vi "E100Backup.vi"() -> ()   [LabVIEW 2012]
uses:
  <vilib>/Utility/NIReport.llb/NI_report.lvclass
  <vilib>/addons/database/Connection.llb/DB Tools Open Connec (Path).vi
  <vilib>/addons/database/Connection.llb/Conn Execute.vi
  <vilib>/addons/database/Recordset.llb/Rec Fetch Recordset Data (R).vi
  <vilib>/addons/database/Recordset.llb/Rec Destroy - Connection.vi
  <vilib>/Utility/NIReport.llb/Append Text Table to Report (wrap).vi
  <vilib>/addons/database/_DB Variant To Data/Database Variant To Data.xnode
  <vilib>/addons/database/NI_Database_API.lvlib
  <vilib>/Utility/NIReport.llb/Excel/NI_Excel.lvclass
  <vilib>/Utility/SMTP/NI_SMTPEmail.lvlib
panel:
  out "data 2":string
  out "data":string
  out "Value":variant
  in  "Table Control 3":string[][](table)
  out "appended array 4":string[](array[string])
  out "error out 5":errorcluster
  in  "Table Control 2":string[][](table)
  out "error out 4":errorcluster
  out "appended array 3":string[](array[string])
  out "recordset data 2":variant[][](array[variant])
  out "recordset data":variant[][](array[variant])
  out "appended array 2":string[](array[string])
  in  "Report Template":path=path "O:/Monitor/Report/E100Backup.xls"
  out "error out 2":errorcluster
  in  "Table Control":string[][](table)
  out "error out 3":errorcluster
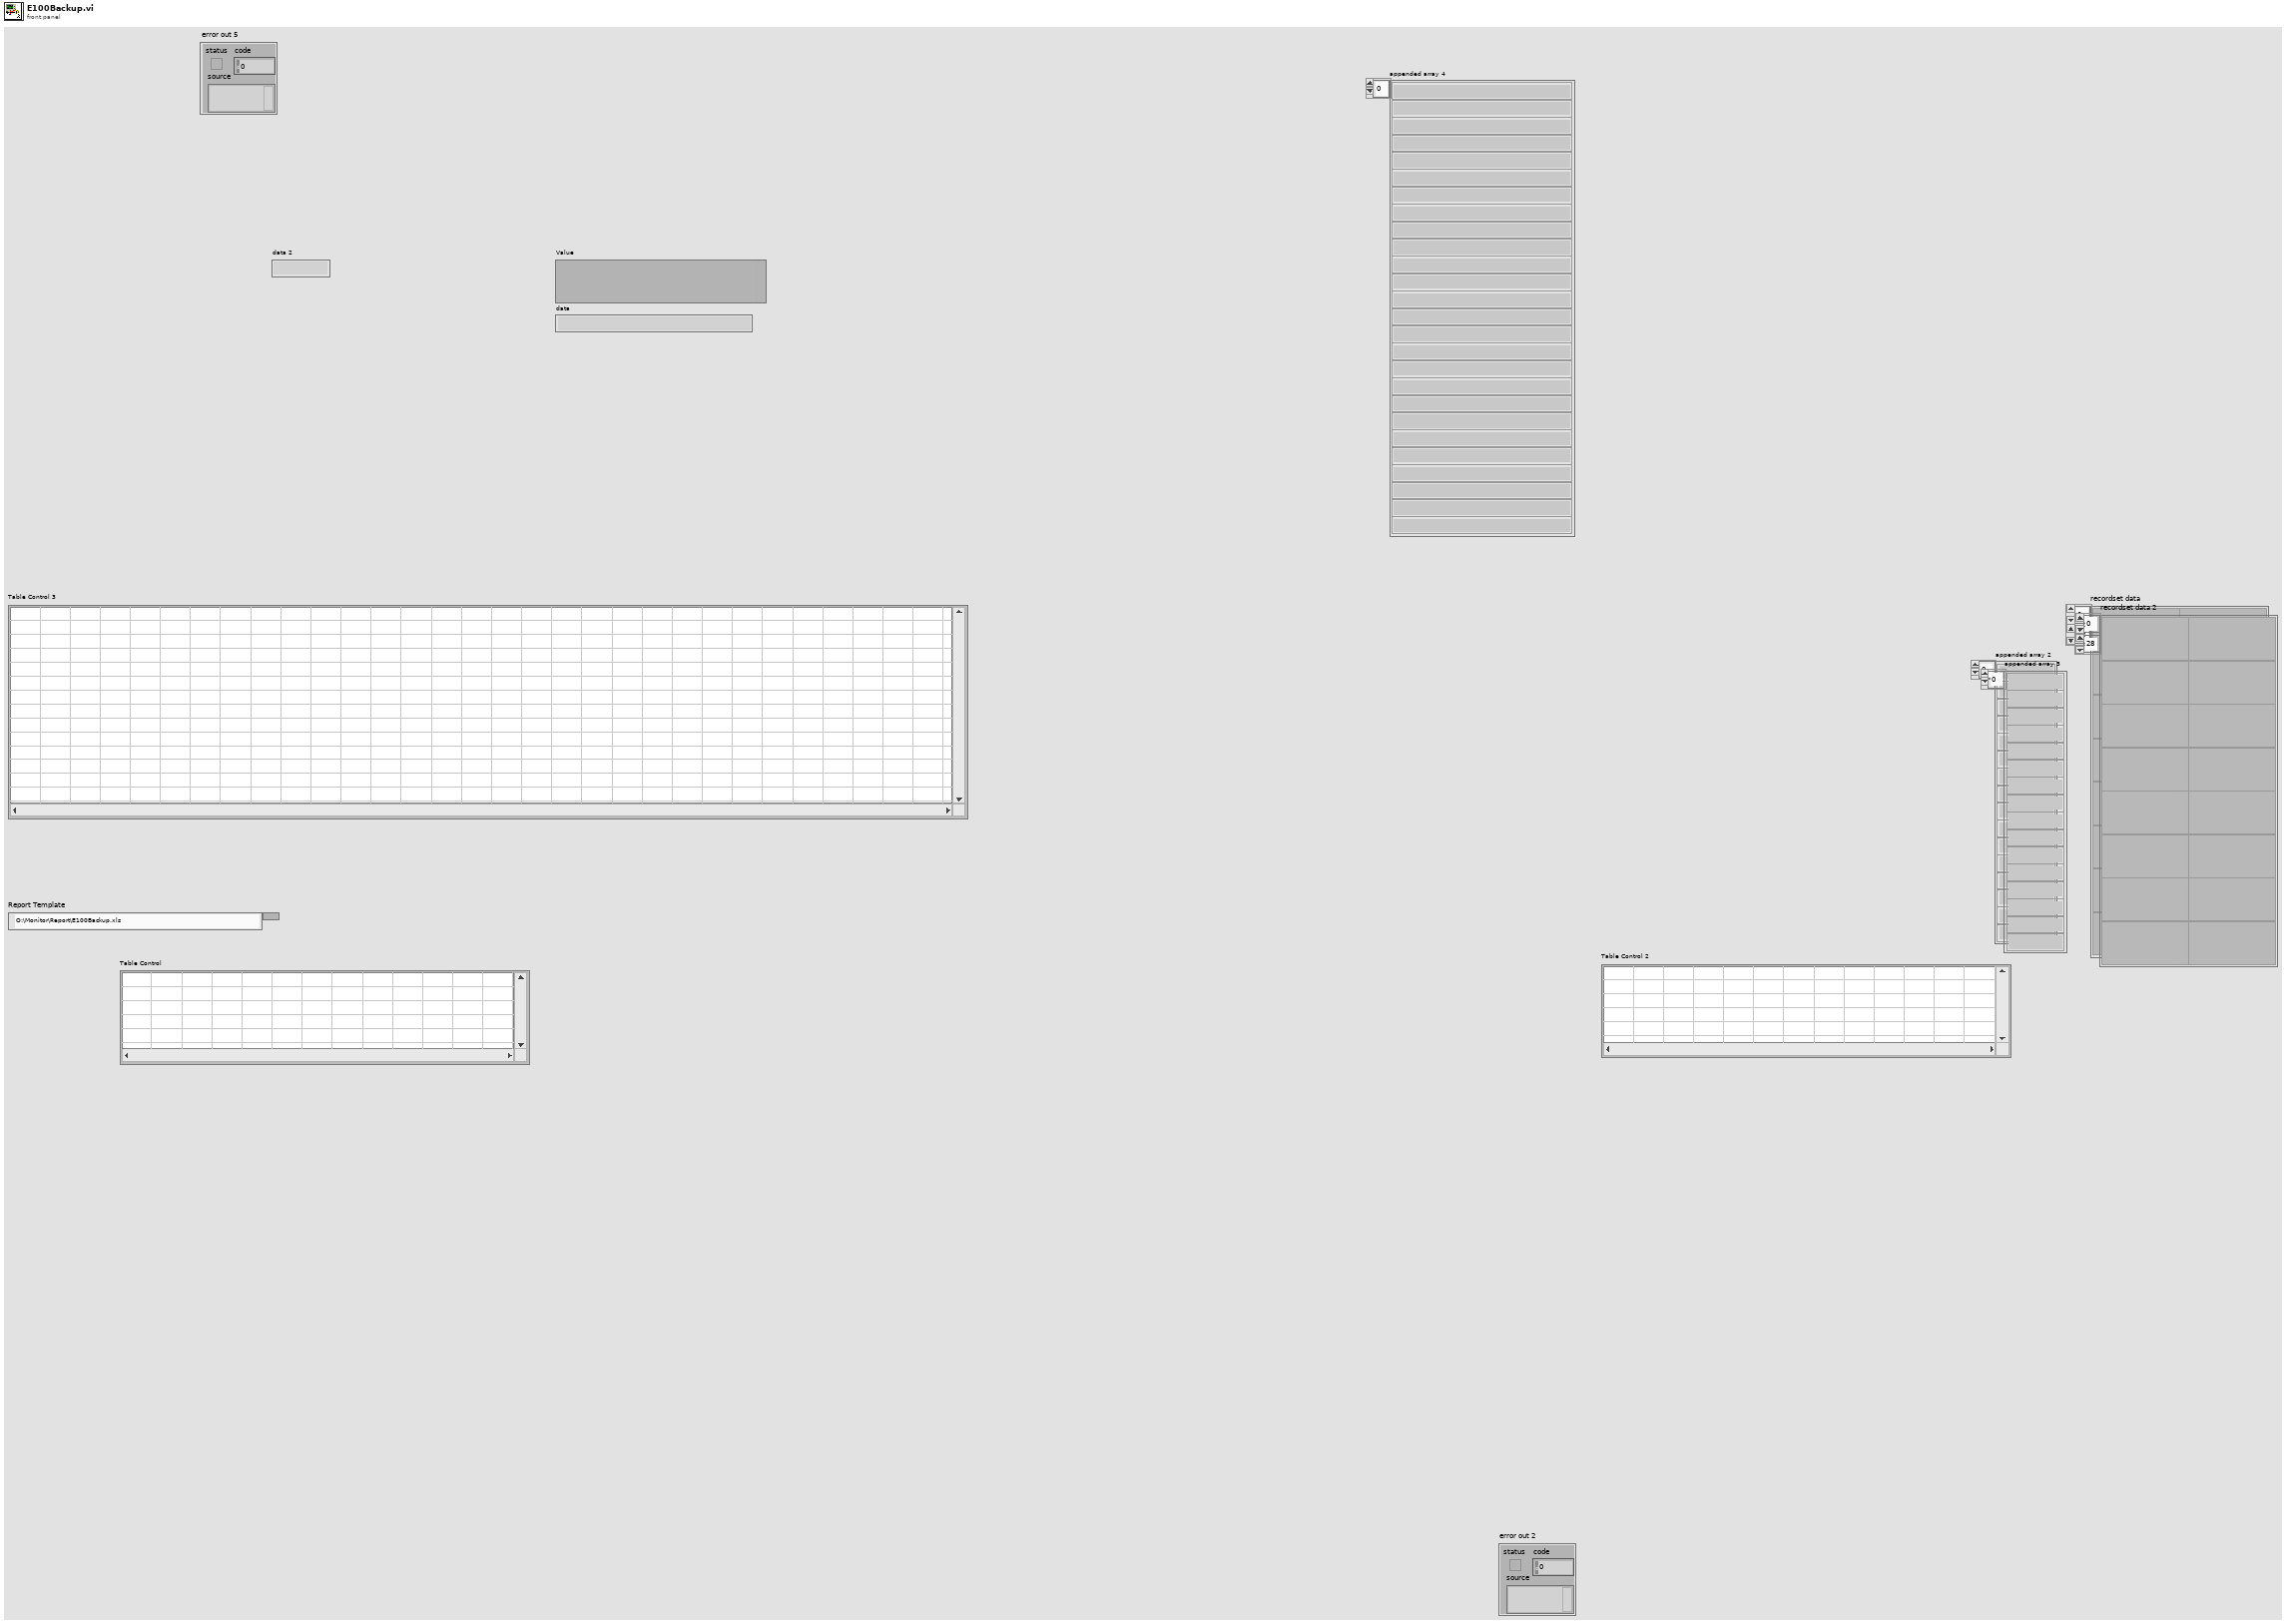
[diagram p1: front panel]
types:
  T1 = typedef "NI_Database_API.lvlib/Conn ObjectReference.ctl" = refnum<k1>
  T2 = typedef "NI_Database_API.lvlib/Rec ObjectReference.ctl" = refnum<k1>
  T3 = enum16{"Standard Report", "HTML", "Word", "Excel"}
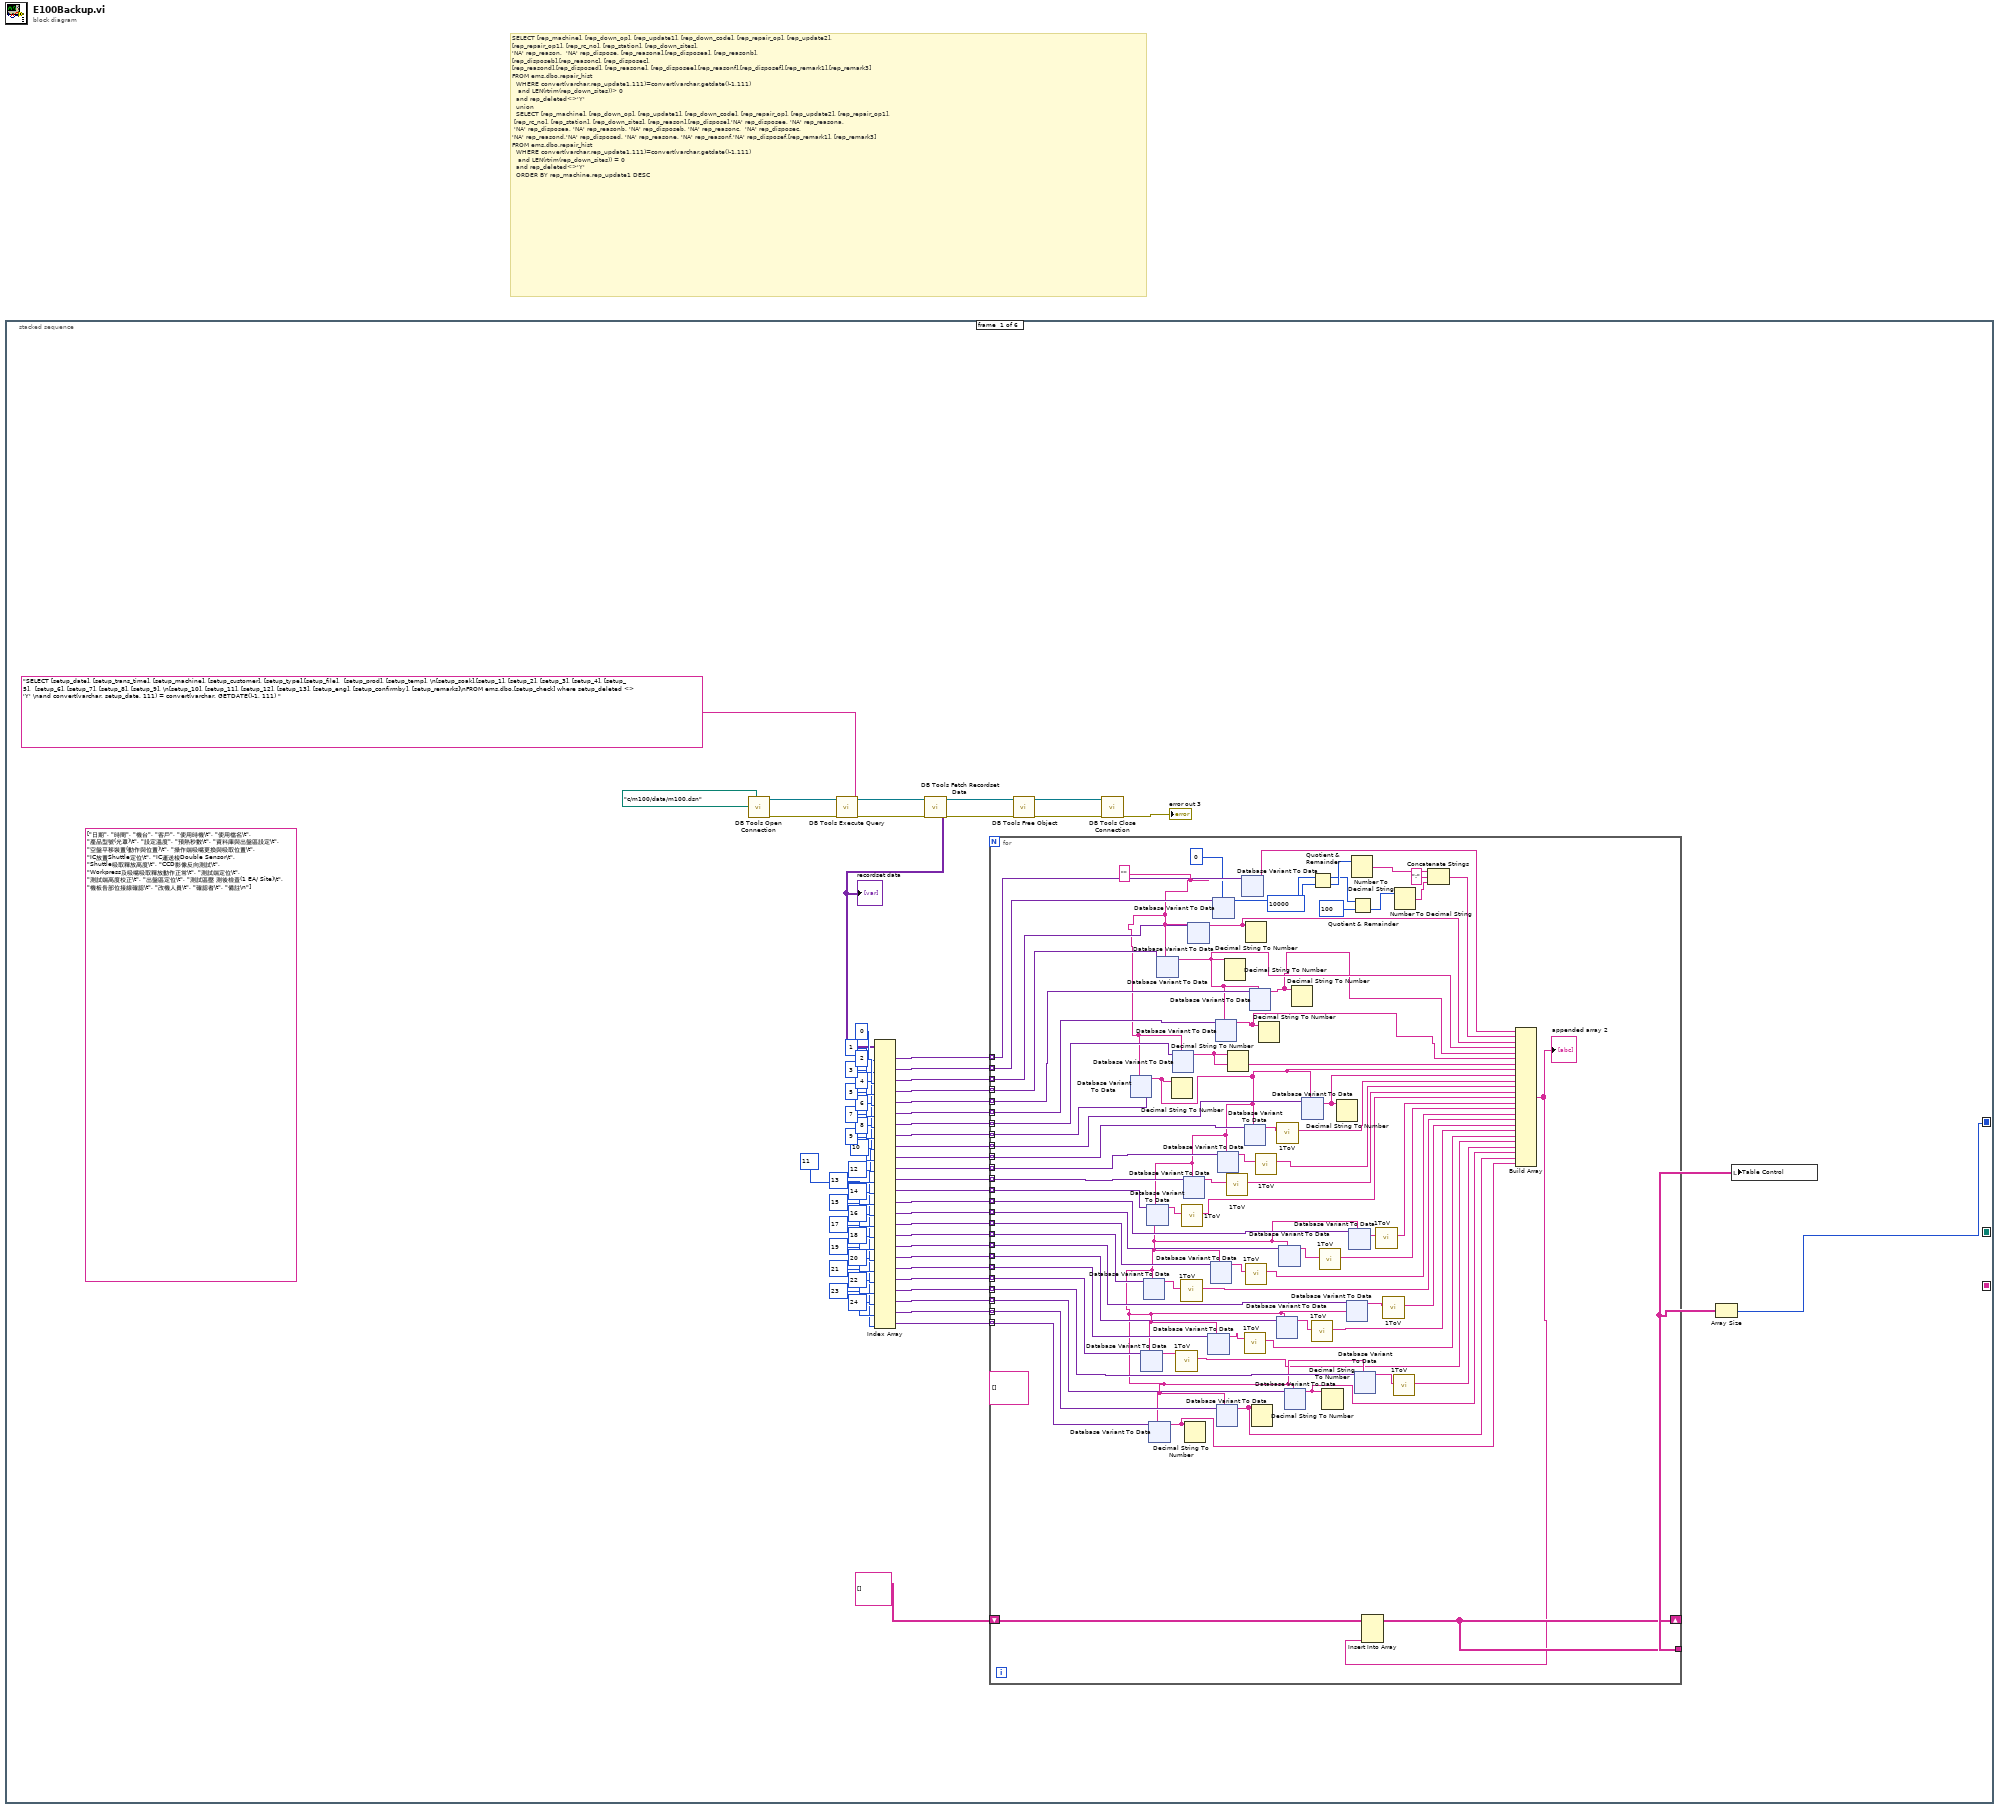
[diagram p0: block diagram]
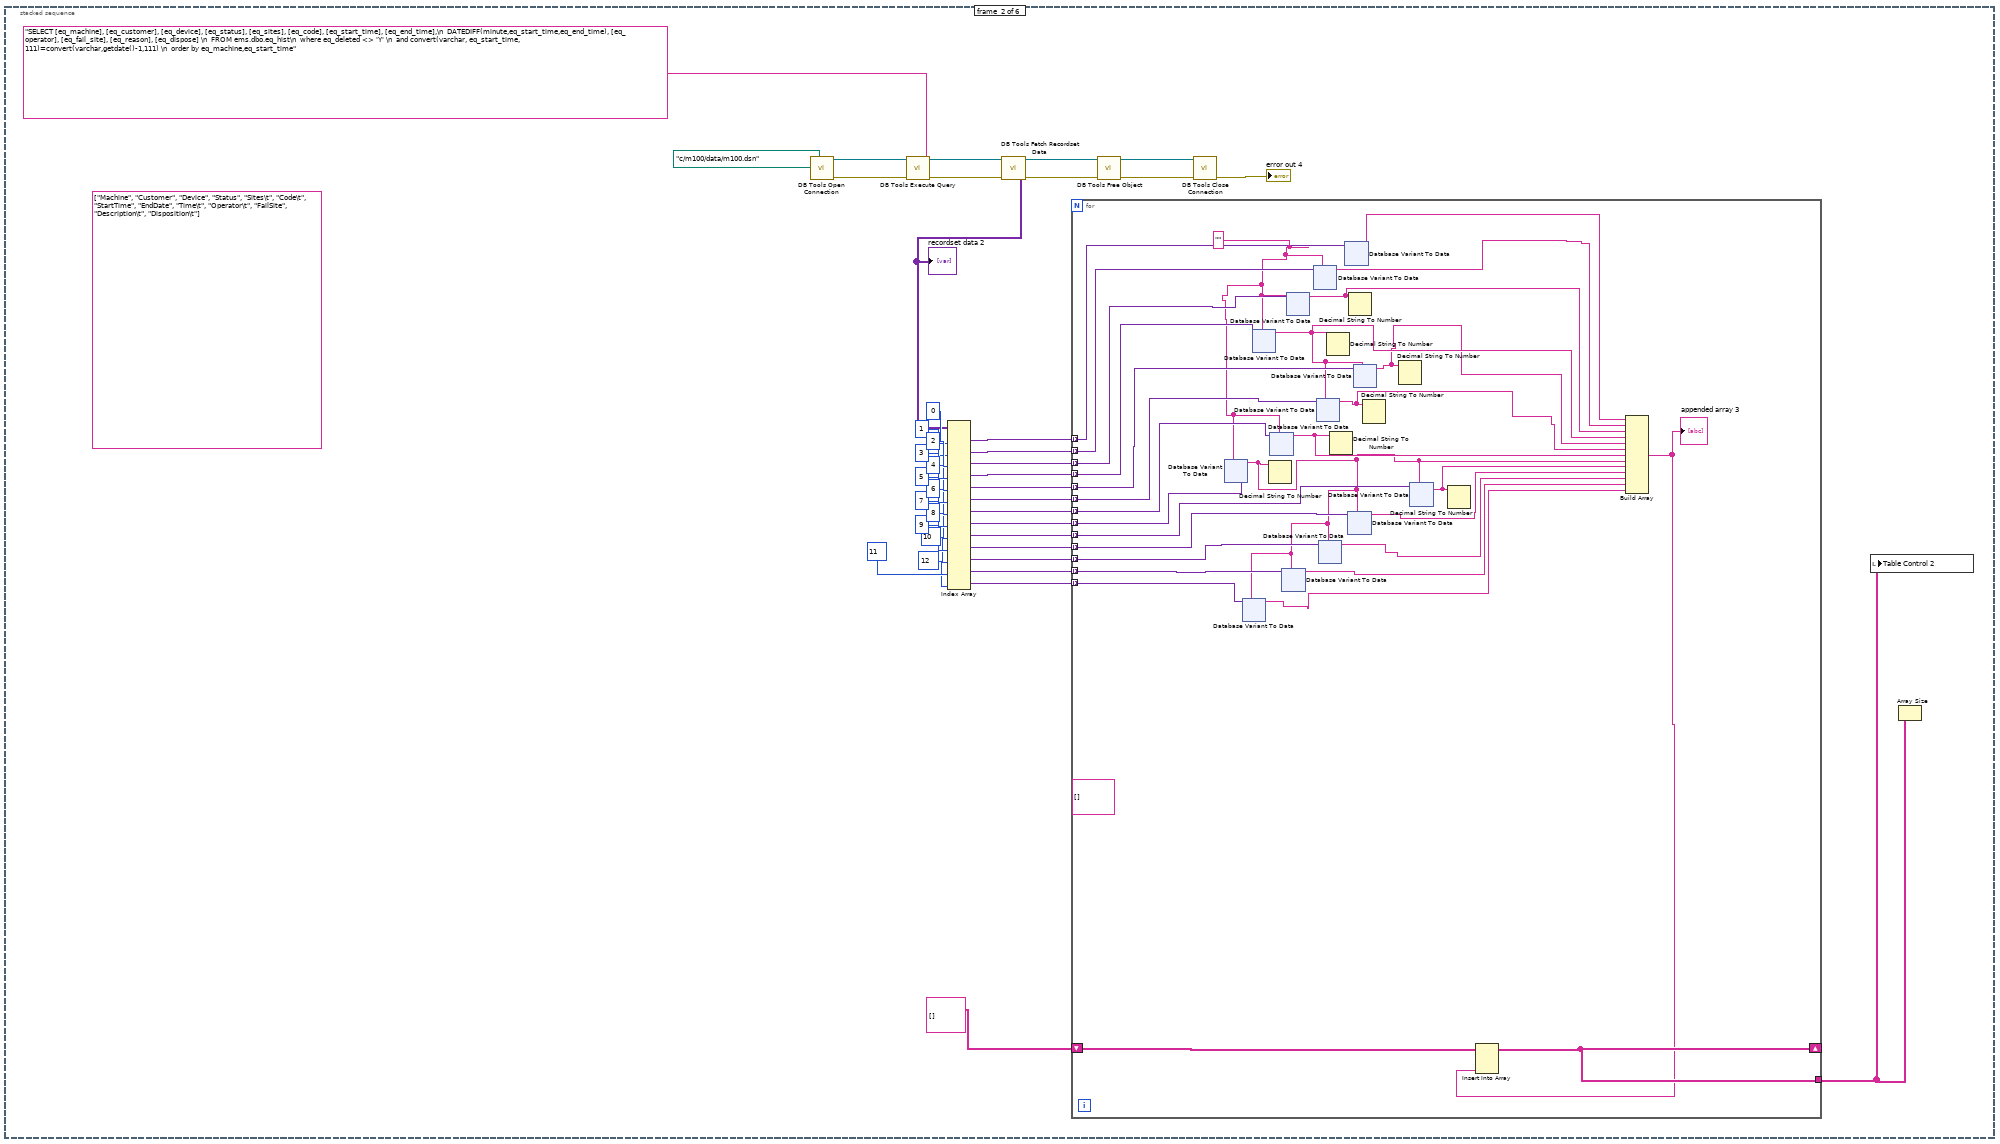
[diagram p2: hidden frame]
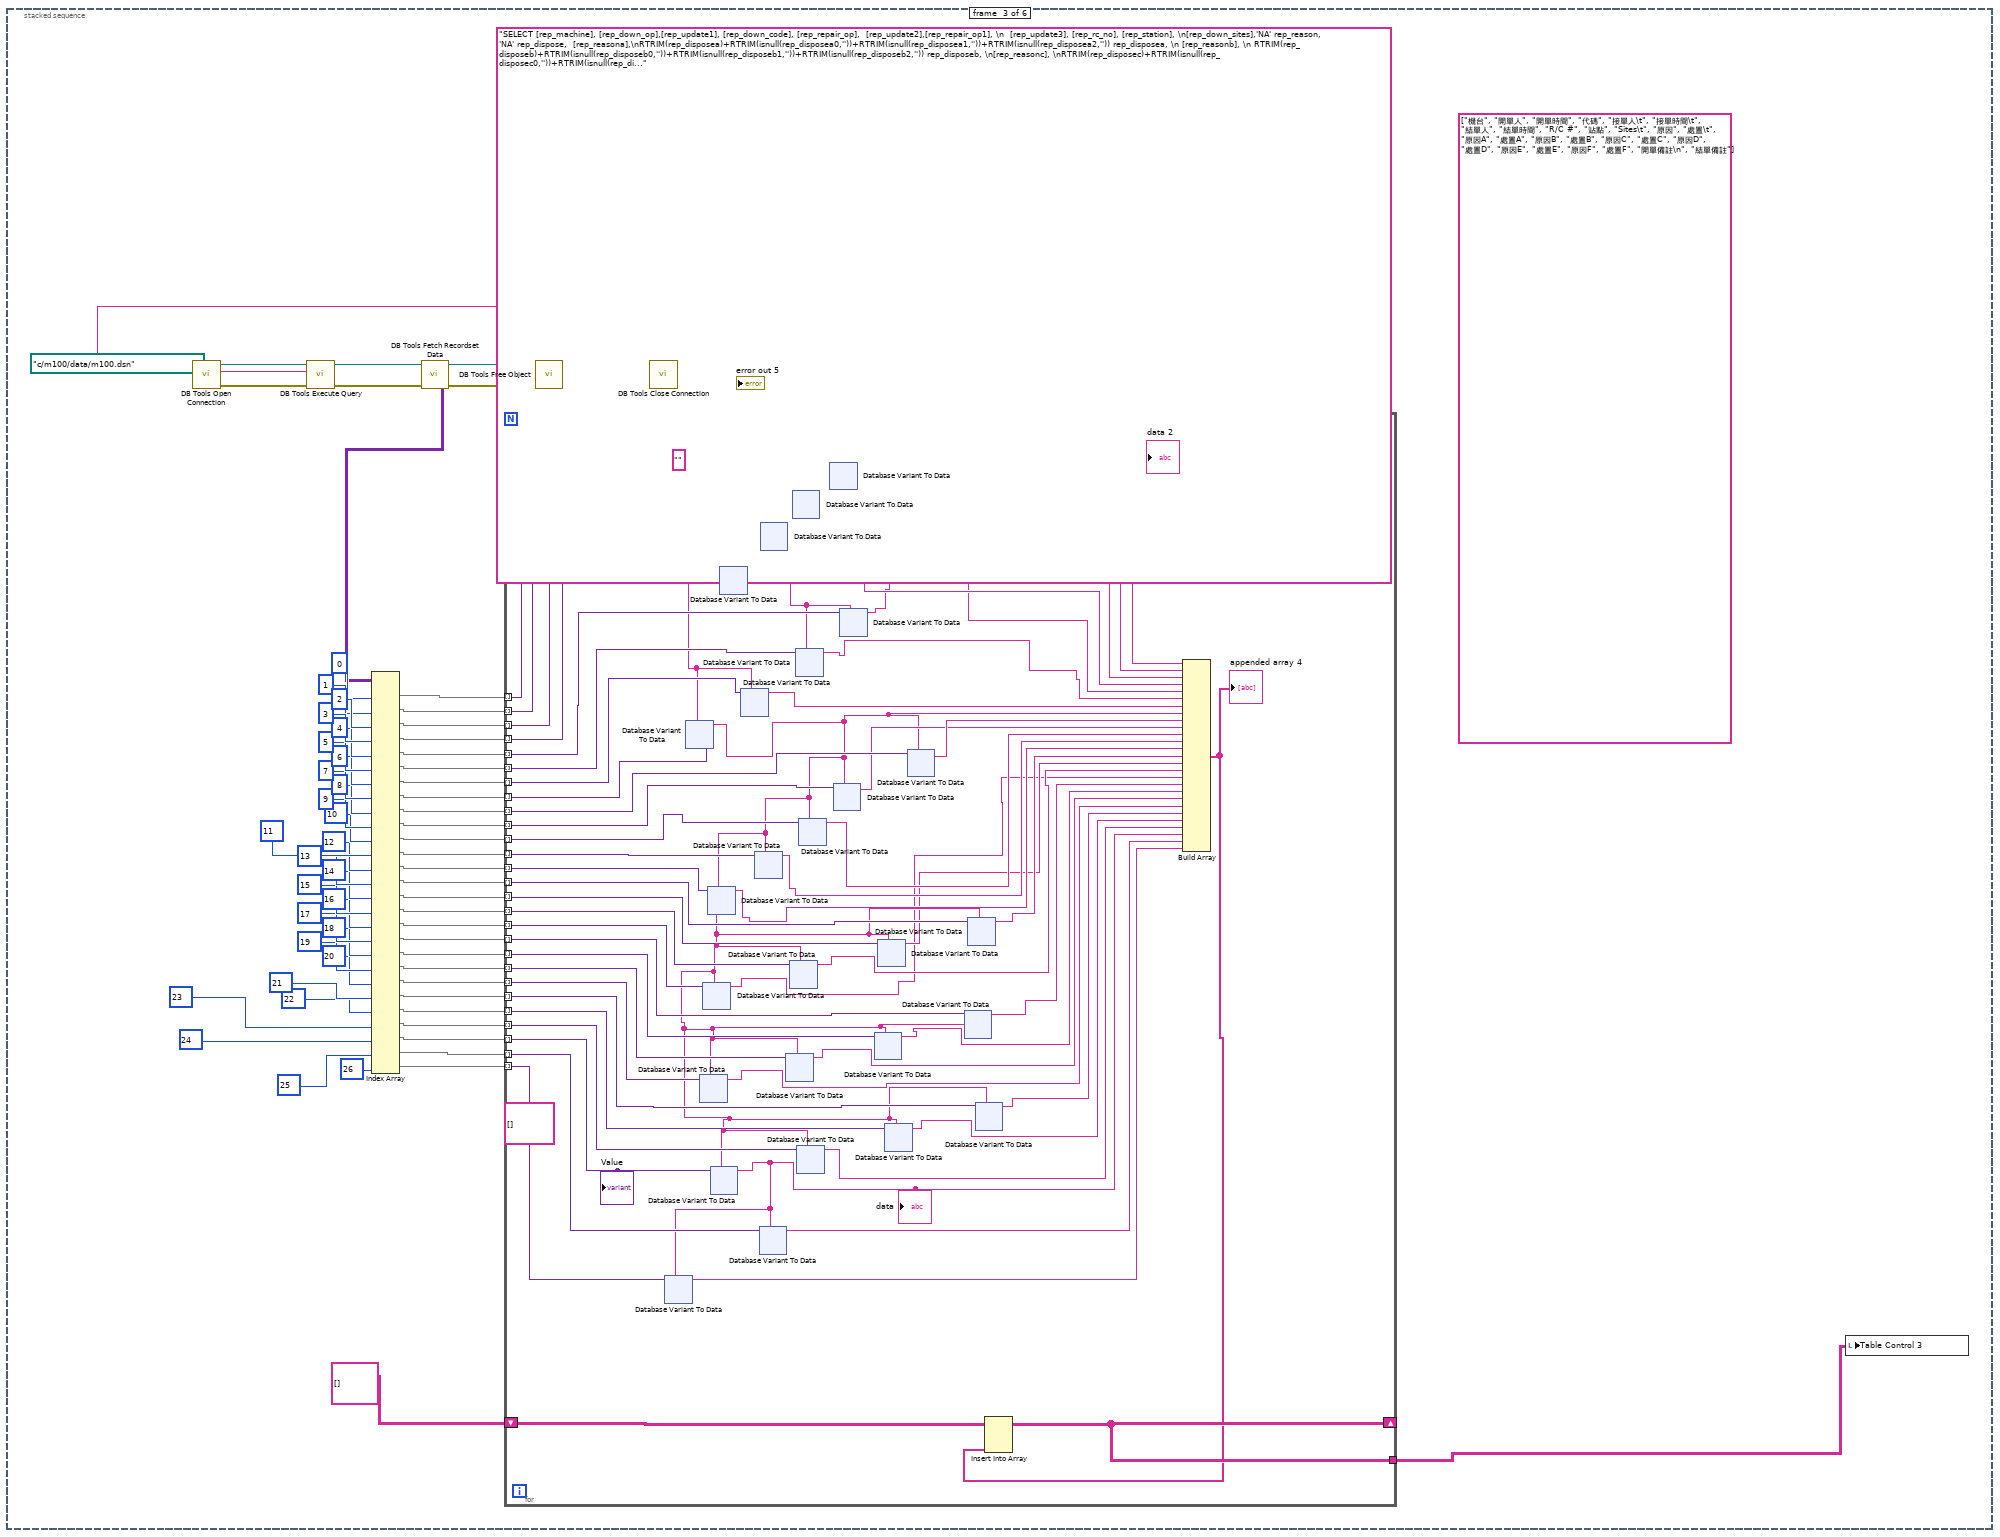
[diagram p3: hidden frame]
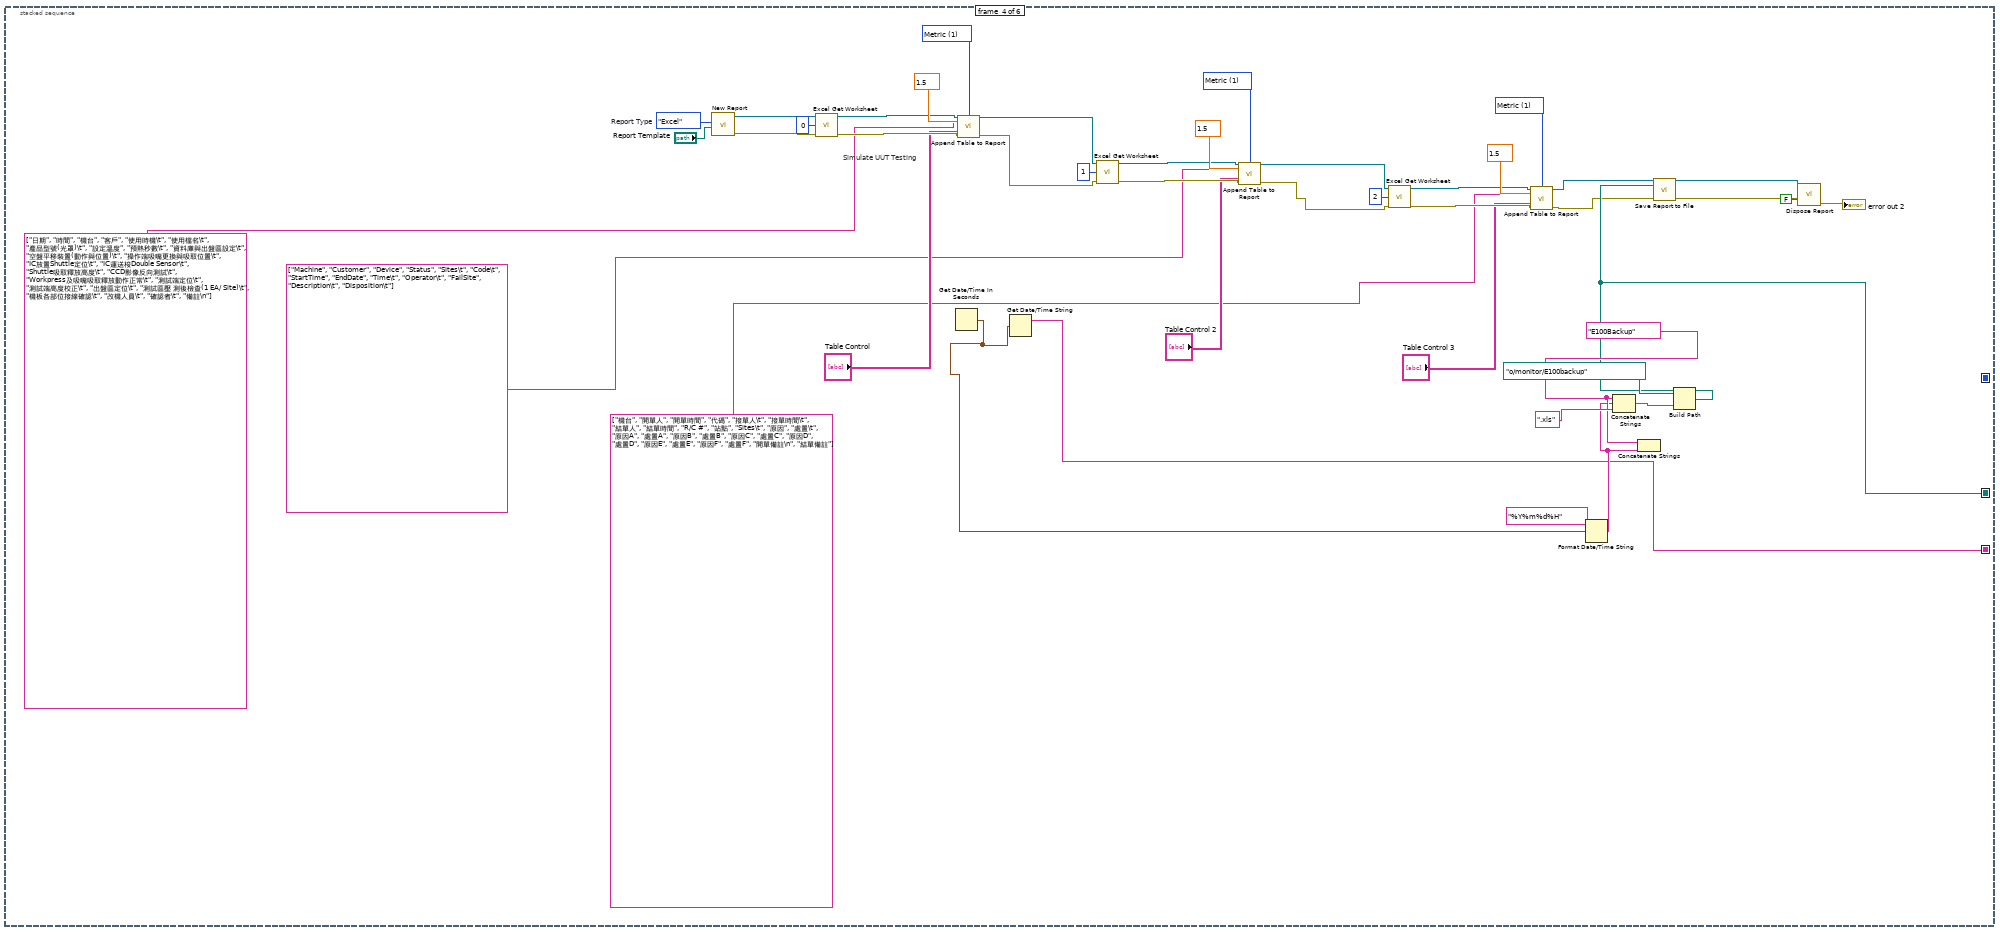
[diagram p4: hidden frame]
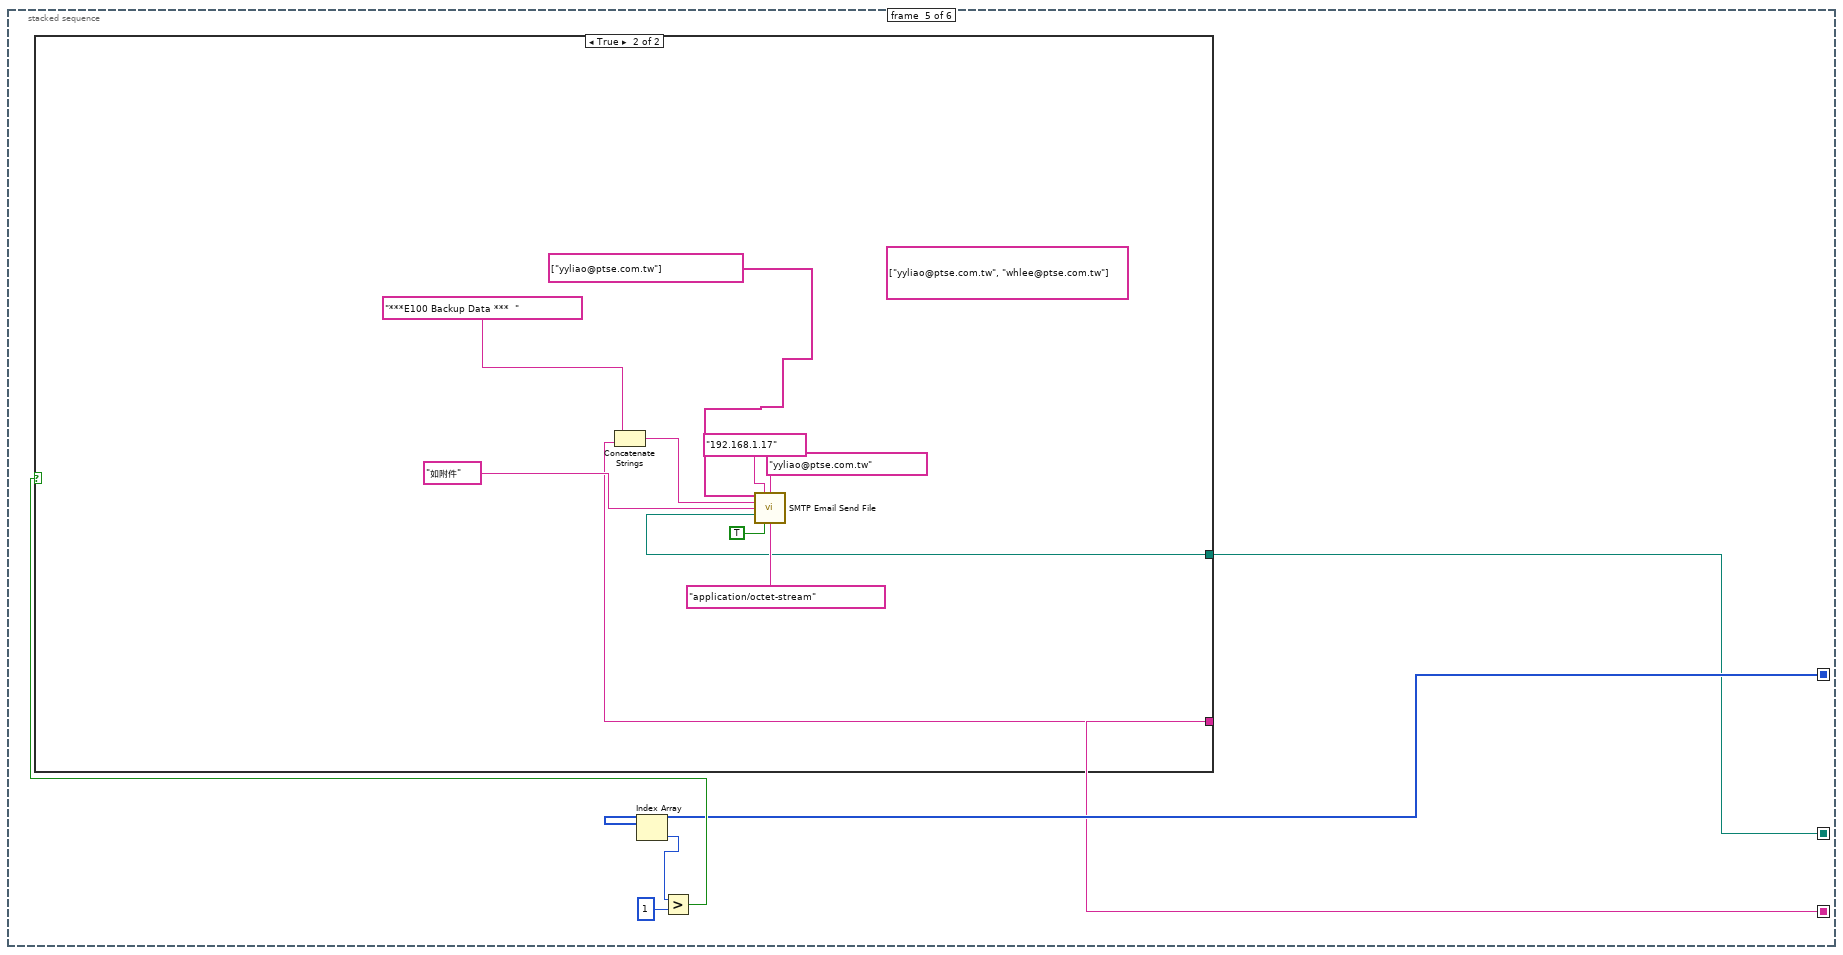
[diagram p5: hidden frame]
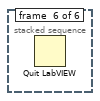
[diagram p7: hidden frame]
diagram:
  # "SELECT [rep_machine], [rep_down_op], [rep_update1], [rep_down_code], [rep_repair_op], [rep_update2], \n[rep_repair_op1], [rep_rc_no], [rep_station], [rep_down_sites], \n'NA' rep_reason,  'NA' rep_dispose, [rep_reasona],[rep_disposea], [rep_reasonb],\n[rep_disposeb],[rep_reasonc], [rep_disposec],\n[rep_reasond],[rep_disposed], [rep_reasone], [rep_disposee],[rep_reasonf],[rep_disposef],[rep_remark1],[rep_remark3] \nFROM ems.dbo.repair_hist \n  WHERE convert(varchar,rep_update1,111)=convert(varchar,getdate()-1,111)\n   and LEN(rtrim(rep_down_sites))> 0 \n  and rep_deleted<>'Y' \n  union\n  SELECT [rep_machine], [rep_down_op], [rep_update1], [rep_down_code], [rep_repair_op], [rep_update2], [rep_repair_op1], \n [rep_rc_no], [rep_station], [rep_down_sites], [rep_reason],[rep_dispose],'NA' rep_disposee, 'NA' rep_reasona,\n 'NA' rep_disposea, 'NA' rep_reasonb, 'NA' rep_disposeb, 'NA' rep_reasonc,  'NA' rep_disposec,\n'NA' rep_reasond,'NA' rep_disposed, 'NA' rep_reasone, 'NA' rep_reasonf,'NA' rep_disposef,[rep_remark1], [rep_remark3] \nFROM ems.dbo.repair_hist \n  WHERE convert(varchar,rep_update1,111)=convert(varchar,getdate()-1,111)\n   and LEN(rtrim(rep_down_sites)) = 0 \n  and rep_deleted<>'Y' \n  ORDER BY rep_machine,rep_update1 DESC"
  n1 = stacked-sequence {
    seq-local: [w54 _ _ _ _ _] -> [_ _ _ _ w2465 _]
    seq-local: [_ _ _ w2443 _ _] -> [_ _ _ _ w2464 _]
    seq-local: [_ _ _ w2441 _ _] -> [_ _ _ _ w2463 _]
    frame #0 {
      (unwired) string[] ["日期", "時間", "機台", "客戶", "使用時機\t", "使用檔名\t", "產品型號(光罩)\t", "設定溫度", "預熱秒數\t", "資料庫與出盤區設定\t", "空盤平移裝置(動作與位置)\t", "操作端吸嘴更換與吸取位置\t", "IC放置Shuttle定位\t", "IC運送梭Double Sensor\t", "Shuttle吸取釋放高度\t", "CCD影像反向測試\t", "Workpress及吸嘴吸取釋放動作正常\t", "測試端定位\t", "測試端高度校正\t", "出盤區定位\t", "測試區壓 測後檢查(1 EA/ Site)\t", "機板各部位接線確認\t", "改機人員\t", "確認者\t", "備註\n"] ("row headers")
      (unwired) string[][] []
      n2 = call-poly <vilib>:"DB Tools Open Connection.vi"("connection information"=path "c:/m100/data/m100.dsn") -> ("error out"=w60:errorcluster, "connection reference"=w64:T1)  [unwired: 7 in]
      n3 = call-poly <vilib>:"DB Tools Execute Query.vi"("error in (no error)"=w60, "SQL query"="SELECT [setup_date], [setup_trans_time], [setup_machine], [setup_customer], [setup_type],[setup_file],  [setup_prod], [setup_temp], \n[setup_soak],[setup_1], [setup_2], [setup_3], [setup_4], [setup_5],  [setup_6], [setup_7], [setup_8], [setup_9], \n[setup_10], [setup_11], [setup_12], [setup_13], [setup_eng], [setup_confirmby], [setup_remarks]\nFROM ems.dbo.[setup_check] where setup_deleted <> 'Y' \nand convert(varchar, setup_date, 111) = convert(varchar, GETDATE()-1, 111) ", "connection reference"=w64) -> ("error out"=w59:errorcluster, "recordset reference"=w63:T2)  [unwired: 5 in]
      n4 = call-poly <vilib>:"DB Tools Fetch Recordset Data.vi"("error in (no error)"=w59, "recordset reference"=w63) -> ("error out"=w58:errorcluster, "recordset data"=w2:variant[][], "recordset reference out"=w62:T2)  [unwired: 3 in]
      "recordset data" <- w2
      n5 = Index Array(array=w2, index (col) #1=0 ("index (row)"), index (col) #2=1 ("index (col)"), index (col) #3=2 ("disabled index (col)"), index (col) #4=3 ("index (col)"), index (col) #5=4 ("index (col)"), index (col) #6=5 ("index (col)"), index (col) #7=6 ("index (col)"), index (col) #8=7 ("index (col)"), index (col) #9=8 ("index (col)"), index (col) #10=9 ("index (col)"), index (col) #11=10 ("index (col)"), index (col) #12=11 ("index (col)"), index (col) #13=12 ("index (col)"), index (col) #14=13 ("index (col)"), index (col) #15=14 ("index (col)"), index (col) #16=15 ("index (col)"), index (col) #17=16 ("index (col)"), index (col) #18=17 ("index (col)"), index (col) #19=18 ("index (col)"), index (col) #20=19 ("index (col)"), index (col) #21=20 ("index (col)"), index (col) #22=21 ("index (col)"), index (col) #23=22 ("index (col)"), index (col) #24=23 ("index (col)"), index (col) #25=24 ("index (col)")) -> (element #1=w32:variant[], element #2=w31:variant[], element #3=w43:variant[], element #4=w42:variant[], element #5=w41:variant[], element #6=w40:variant[], element #7=w39:variant[], element #8=w38:variant[], element #9=w37:variant[], element #10=w36:variant[], element #11=w35:variant[], element #12=w34:variant[], element #13=w15:variant[], element #14=w14:variant[], element #15=w13:variant[], element #16=w12:variant[], element #17=w11:variant[], element #18=w10:variant[], element #19=w9:variant[], element #20=w8:variant[], element #21=w7:variant[], element #22=w6:variant[], element #23=w5:variant[], element #24=w4:variant[], element #25=w3:variant[])  [unwired: 25 in]
      n6 = for {
        tunnel: w43 -> [w138] mode=indexing
        tunnel: w42 -> [w137] mode=indexing
        tunnel: w41 -> [w136] mode=indexing
        tunnel: w40 -> [w135] mode=indexing
        tunnel: w39 -> [w134] mode=indexing
        tunnel: w38 -> [w133] mode=indexing
        tunnel: w37 -> [w132] mode=indexing
        tunnel: w36 -> [w131] mode=indexing
        tunnel: w35 -> [w130] mode=indexing
        tunnel: w34 -> [w129] mode=indexing
        tunnel: [w142] -> w1
        shift-right: [w142] -> _
        shift-left: string[][] [] ("array") -> [w141]
        tunnel: w32 -> [w140] mode=indexing
        tunnel: w31 -> [w139] mode=indexing
        tunnel: w15 -> [w127] mode=indexing
        tunnel: w14 -> [w126] mode=indexing
        tunnel: w13 -> [w125] mode=indexing
        tunnel: w12 -> [w124] mode=indexing
        tunnel: w11 -> [w123] mode=indexing
        tunnel: w10 -> [w122] mode=indexing
        tunnel: w9 -> [w119] mode=indexing
        tunnel: w8 -> [w121] mode=indexing
        tunnel: w7 -> [w120] mode=indexing
        tunnel: w6 -> [w118] mode=indexing
        tunnel: w5 -> [w117] mode=indexing
        tunnel: w4 -> [w115] mode=indexing
        tunnel: w3 -> [w116] mode=indexing
        w111 = ""
        n7 = xnode "Database Variant To Data"("database variant"=w133, "type"=w111) -> ("data"=w108:string)  [unwired: 1 in, 1 out]
        n8 = xnode "Database Variant To Data"("database variant"=w127, "type"=w108) -> ("data"=w85:string)  [unwired: 1 in, 1 out]
        n9 = xnode "Database Variant To Data"("database variant"=w120, "type"=w85) -> ("data"=w69:string)  [unwired: 1 in, 1 out]
        n10 = xnode "Database Variant To Data"("database variant"=w123, "type"=w85) -> ("data"=w77:string)  [unwired: 1 in, 1 out]
        n11 = xnode "Database Variant To Data"("database variant"=w116, "type"=w85) -> ("data"=w105:string)  [unwired: 1 in, 1 out]
        n12 = xnode "Database Variant To Data"("database variant"=w137, "type"=w111) -> ("data"=w114:string)  [unwired: 1 in, 1 out]
        n13 = Decimal String To Number(string=w108) -> ()  [unwired: 2 in, 2 out]
        n14 = xnode "Database Variant To Data"("database variant"=w134, "type"=w111) -> ("data"=w110:string)  [unwired: 1 in, 1 out]
        n15 = call "1ToV.vi"("In1"=w69) -> ("OutV"=w68:string)  [unwired: 10 in]
        n16 = call "1ToV.vi"("In1"=w77) -> ("OutV"=w76:string)  [unwired: 10 in]
        n17 = call "1ToV.vi"("In1"=w85) -> ("OutV"=w84:string)  [unwired: 10 in]
        n18 = xnode "Database Variant To Data"("database variant"=w129, "type"=w108) -> ("data"=w88:string)  [unwired: 1 in, 1 out]
        n19 = Decimal String To Number(string=w105) -> ()  [unwired: 2 in, 2 out]
        n20 = xnode "Database Variant To Data"("database variant"=w138, "type"=w111) -> ("data"=w104:string)  [unwired: 1 in, 1 out]
        n21 = xnode "Database Variant To Data"("database variant"=w121, "type"=w85) -> ("data"=w71:string)  [unwired: 1 in, 1 out]
        n22 = xnode "Database Variant To Data"("database variant"=w124, "type"=w85) -> ("data"=w79:string)  [unwired: 1 in, 1 out]
        n23 = xnode "Database Variant To Data"("database variant"=w139, "type"=0) -> ("data"=w101:i32)  [unwired: 1 in, 1 out]
        n24 = xnode "Database Variant To Data"("database variant"=w135, "type"=w114) -> ("data"=w112:string)  [unwired: 1 in, 1 out]
        n25 = xnode "Database Variant To Data"("database variant"=w115, "type"=w85) -> ("data"=w106:string)  [unwired: 1 in, 1 out]
        n26 = xnode "Database Variant To Data"("database variant"=w130, "type"=w108) -> ("data"=w91:string)  [unwired: 1 in, 1 out]
        n27 = Decimal String To Number(string=w114) -> ()  [unwired: 2 in, 2 out]
        n28 = call "1ToV.vi"("In1"=w88) -> ("OutV"=w86:string)  [unwired: 10 in]
        n29 = Decimal String To Number(string=w110) -> ()  [unwired: 2 in, 2 out]
        n30 = xnode "Database Variant To Data"("database variant"=w140, "type"=w111) -> ("data"=w103:string)  [unwired: 1 in, 1 out]
        n31 = xnode "Database Variant To Data"("database variant"=w131, "type"=w108) -> ("data"=w90:string)  [unwired: 1 in, 1 out]
        n32 = call "1ToV.vi"("In1"=w71) -> ("OutV"=w70:string)  [unwired: 10 in]
        n33 = Decimal String To Number(string=w104) -> ()  [unwired: 2 in, 2 out]
        n34 = call "1ToV.vi"("In1"=w79) -> ("OutV"=w78:string)  [unwired: 10 in]
        n35 = xnode "Database Variant To Data"("database variant"=w136, "type"=w114) -> ("data"=w113:string)  [unwired: 1 in, 1 out]
        n36 = Decimal String To Number(string=w106) -> ()  [unwired: 2 in, 2 out]
        n37 = call "1ToV.vi"("In1"=w91) -> ("OutV"=w87:string)  [unwired: 10 in]
        n38 = Decimal String To Number(string=w112) -> ()  [unwired: 2 in, 2 out]
        n39 = xnode "Database Variant To Data"("database variant"=w119, "type"=w85) -> ("data"=w73:string)  [unwired: 1 in, 1 out]
        n40 = call "1ToV.vi"("In1"=w90) -> ("OutV"=w89:string)  [unwired: 10 in]
        n41 = xnode "Database Variant To Data"("database variant"=w125, "type"=w85) -> ("data"=w82:string)  [unwired: 1 in, 1 out]
        n42 = xnode "Database Variant To Data"("database variant"=w117, "type"=w85) -> ("data"=w107:string)  [unwired: 1 in, 1 out]
        n43 = Decimal String To Number(string=w113) -> ()  [unwired: 2 in, 2 out]
        n44 = xnode "Database Variant To Data"("database variant"=w132, "type"=w108) -> ("data"=w109:string)  [unwired: 1 in, 1 out]
        n45 = call "1ToV.vi"("In1"=w73) -> ("OutV"=w72:string)  [unwired: 10 in]
        n46 = Quotient & Remainder(x=w101, y=10000) -> (x-y*floor(x/y)=w92:i32, floor(x/y)=w93:i32)
        n47 = call "1ToV.vi"("In1"=w82) -> ("OutV"=w80:string)  [unwired: 10 in]
        n48 = Decimal String To Number(string=w107) -> ()  [unwired: 2 in, 2 out]
        n49 = Decimal String To Number(string=w109) -> ()  [unwired: 2 in, 2 out]
        n50 = xnode "Database Variant To Data"("database variant"=w122, "type"=w85) -> ("data"=w75:string)  [unwired: 1 in, 1 out]
        n51 = xnode "Database Variant To Data"("database variant"=w126, "type"=w85) -> ("data"=w83:string)  [unwired: 1 in, 1 out]
        n52 = Number To Decimal String(number=w93) -> (decimal integer string=w98:string)  [unwired: 1 in]
        n53 = Quotient & Remainder(x=w92, y=100) -> (floor(x/y)=w94:i32)  [unwired: 1 out]
        n54 = xnode "Database Variant To Data"("database variant"=w118, "type"=w85) -> ("data"=w67:string)  [unwired: 1 in, 1 out]
        n55 = call "1ToV.vi"("In1"=w83) -> ("OutV"=w81:string)  [unwired: 10 in]
        n56 = call "1ToV.vi"("In1"=w75) -> ("OutV"=w74:string)  [unwired: 10 in]
        n57 = call "1ToV.vi"("In1"=w67) -> ("OutV"=w66:string)  [unwired: 10 in]
        n58 = Number To Decimal String(number=w94) -> (decimal integer string=w96:string)  [unwired: 1 in]
        n59 = Concatenate Strings(w98, ":" ("string"), w96) -> (w95:string)
        n60 = Build Array(w103, w95, w104, w114, w113, w112, w110, w108, w109, w89, w87, w86, w84, w81, w80, w78, w76, w74, w72, w70, w68, w66, w107, w106, w105) -> (w128:string[])
        "appended array 2" <- w128
        n61 = Insert Into Array(array=w141, new element=w128) -> (w142:string[][])  [unwired: 2 in]
      }
      n62 = call-poly <vilib>:"DB Tools Free Object.vi"("error in (no error)"=w58, "recordset reference"=w62) -> ("error out"=w57:errorcluster, "connection reference"=w61:T1)  [unwired: 8 in]
      n63 = call <vilib>:"DB Tools Close Connection.vi"("error in (no error)"=w57, "connection reference"=w61) -> ("error out"=→"error out 3":errorcluster)  [unwired: 5 in]
      n64 = Array Size(array=w1) -> (size(s)=w54:i32[])
      n65 = local write "Table Control"(w1) -> ()
    }
    frame #1 {
      (unwired) string[] ["Machine", "Customer", "Device", "Status", "Sites\t", "Code\t", "StartTime", "EndDate", "Time\t", "Operator\t", "FailSite", "Description\t", "Disposition\t"] ("row headers")
      (unwired) string[][] []
      n66 = call-poly <vilib>:"DB Tools Open Connection.vi"("connection information"=path "c:/m100/data/m100.dsn") -> ("error out"=w977:errorcluster, "connection reference"=w981:T1)  [unwired: 7 in]
      n67 = call-poly <vilib>:"DB Tools Execute Query.vi"("error in (no error)"=w977, "SQL query"="SELECT [eq_machine], [eq_customer], [eq_device], [eq_status], [eq_sites], [eq_code], [eq_start_time], [eq_end_time],\n  DATEDIFF(minute,eq_start_time,eq_end_time), [eq_operator], [eq_fail_site], [eq_reason], [eq_dispose] \n  FROM ems.dbo.eq_hist\n  where eq_deleted <> 'Y' \n  and convert(varchar, eq_start_time, 111)=convert(varchar,getdate()-1,111) \n  order by eq_machine,eq_start_time", "connection reference"=w981) -> ("error out"=w976:errorcluster, "recordset reference"=w980:T2)  [unwired: 5 in]
      n68 = call-poly <vilib>:"DB Tools Fetch Recordset Data.vi"("error in (no error)"=w976, "recordset reference"=w980) -> ("error out"=w975:errorcluster, "recordset data"=w944:variant[][], "recordset reference out"=w979:T2)  [unwired: 3 in]
      "recordset data 2" <- w944
      n69 = Index Array(array=w944, index (col) #1=0 ("index (row)"), index (col) #2=1 ("index (col)"), index (col) #3=2 ("disabled index (col)"), index (col) #4=3 ("index (col)"), index (col) #5=4 ("index (col)"), index (col) #6=5 ("index (col)"), index (col) #7=6 ("index (col)"), index (col) #8=7 ("index (col)"), index (col) #9=8 ("index (col)"), index (col) #10=9 ("index (col)"), index (col) #11=10 ("index (col)"), index (col) #12=11 ("index (col)"), index (col) #13=12 ("index (col)")) -> (element #1=w950:variant[], element #2=w949:variant[], element #3=w961:variant[], element #4=w960:variant[], element #5=w959:variant[], element #6=w958:variant[], element #7=w957:variant[], element #8=w956:variant[], element #9=w955:variant[], element #10=w954:variant[], element #11=w953:variant[], element #12=w952:variant[], element #13=w945:variant[])  [unwired: 13 in]
      n70 = for {
        tunnel: w961 -> [w1008] mode=indexing
        tunnel: w960 -> [w1007] mode=indexing
        tunnel: w959 -> [w1006] mode=indexing
        tunnel: w958 -> [w1005] mode=indexing
        tunnel: w957 -> [w1004] mode=indexing
        tunnel: w956 -> [w1003] mode=indexing
        tunnel: w955 -> [w1002] mode=indexing
        tunnel: w954 -> [w1001] mode=indexing
        tunnel: w953 -> [w1000] mode=indexing
        tunnel: w952 -> [w999] mode=indexing
        tunnel: [w1012] -> w943
        shift-right: [w1012] -> _
        shift-left: string[][] [] ("array") -> [w1011]
        tunnel: w950 -> [w1010] mode=indexing
        tunnel: w949 -> [w1009] mode=indexing
        tunnel: w945 -> [w997] mode=indexing
        w983 = ""
        n71 = xnode "Database Variant To Data"("database variant"=w1003, "type"=w983) -> ("data"=w991:string)  [unwired: 1 in, 1 out]
        n72 = xnode "Database Variant To Data"("database variant"=w997, "type"=w991) -> ("data"=w985:string)  [unwired: 1 in, 1 out]
        n73 = xnode "Database Variant To Data"("database variant"=w1007, "type"=w983) -> ("data"=w996:string)  [unwired: 1 in, 1 out]
        n74 = Decimal String To Number(string=w991) -> ()  [unwired: 2 in, 2 out]
        n75 = xnode "Database Variant To Data"("database variant"=w1004, "type"=w983) -> ("data"=w993:string)  [unwired: 1 in, 1 out]
        n76 = xnode "Database Variant To Data"("database variant"=w999, "type"=w991) -> ("data"=w986:string)  [unwired: 1 in, 1 out]
        n77 = xnode "Database Variant To Data"("database variant"=w1008, "type"=w983) -> ("data"=w990:string)  [unwired: 1 in, 1 out]
        n78 = xnode "Database Variant To Data"("database variant"=w1009, "type"=w983) -> ("data"=w984:string)  [unwired: 1 in, 1 out]
        n79 = xnode "Database Variant To Data"("database variant"=w1005, "type"=w996) -> ("data"=w994:string)  [unwired: 1 in, 1 out]
        n80 = xnode "Database Variant To Data"("database variant"=w1000, "type"=w991) -> ("data"=w987:string)  [unwired: 1 in, 1 out]
        n81 = Decimal String To Number(string=w996) -> ()  [unwired: 2 in, 2 out]
        n82 = Decimal String To Number(string=w993) -> ()  [unwired: 2 in, 2 out]
        n83 = xnode "Database Variant To Data"("database variant"=w1010, "type"=w983) -> ("data"=w989:string)  [unwired: 1 in, 1 out]
        n84 = xnode "Database Variant To Data"("database variant"=w1001, "type"=w991) -> ("data"=w988:string)  [unwired: 1 in, 1 out]
        n85 = Decimal String To Number(string=w990) -> ()  [unwired: 2 in, 2 out]
        n86 = xnode "Database Variant To Data"("database variant"=w1006, "type"=w996) -> ("data"=w995:string)  [unwired: 1 in, 1 out]
        n87 = Decimal String To Number(string=w994) -> ()  [unwired: 2 in, 2 out]
        n88 = Decimal String To Number(string=w995) -> ()  [unwired: 2 in, 2 out]
        n89 = xnode "Database Variant To Data"("database variant"=w1002, "type"=w991) -> ("data"=w992:string)  [unwired: 1 in, 1 out]
        n90 = Decimal String To Number(string=w992) -> ()  [unwired: 2 in, 2 out]
        n91 = Build Array(w989, w984, w990, w996, w995, w994, w993, w991, w992, w988, w987, w986, w985) -> (w998:string[])
        "appended array 3" <- w998
        n92 = Insert Into Array(array=w1011, new element=w998) -> (w1012:string[][])  [unwired: 2 in]
      }
      n93 = call-poly <vilib>:"DB Tools Free Object.vi"("error in (no error)"=w975, "recordset reference"=w979) -> ("error out"=w974:errorcluster, "connection reference"=w978:T1)  [unwired: 8 in]
      n94 = call <vilib>:"DB Tools Close Connection.vi"("error in (no error)"=w974, "connection reference"=w978) -> ("error out"=→"error out 4":errorcluster)  [unwired: 5 in]
      n95 = local write "Table Control 2"(w943) -> ()
      n96 = Array Size(array=w943) -> ()  [unwired: 1 out]
    }
    frame #2 {
      (unwired) string[] ["機台", "開單人", "開單時間", "代碼", "接單人\t", "接單時間\t", "結單人", "結單時間", "R/C #", "站點", "Sites\t", "原因", "處置\t", "原因A", "處置A", "原因B", "處置B", "原因C", "處置C", "原因D", "處置D", "原因E", "處置E", "原因F", "處置F", "開單備註\n", "結單備註"] ("row headers")
      (unwired) string[][] []
      n97 = call-poly <vilib>:"DB Tools Open Connection.vi"("connection information"=path "c:/m100/data/m100.dsn") -> ("error out"=w1491:errorcluster, "connection reference"=w1495:T1)  [unwired: 7 in]
      n98 = call-poly <vilib>:"DB Tools Execute Query.vi"("error in (no error)"=w1491, "SQL query"="SELECT [rep_machine], [rep_down_op],[rep_update1], [rep_down_code], [rep_repair_op],  [rep_update2],[rep_repair_op1], \n  [rep_update3], [rep_rc_no], [rep_station], \n[rep_down_sites],'NA' rep_reason, 'NA' rep_dispose,  [rep_reasona],\nRTRIM(rep_disposea)+RTRIM(isnull(rep_disposea0,''))+RTRIM(isnull(rep_disposea1,''))+RTRIM(isnull(rep_disposea2,'')) rep_disposea, \n [rep_reasonb], \n RTRIM(rep_disposeb)+RTRIM(isnull(rep_disposeb0,''))+RTRIM(isnull(rep_disposeb1,''))+RTRIM(isnull(rep_disposeb2,'')) rep_disposeb, \n[rep_reasonc], \nRTRIM(rep_disposec)+RTRIM(isnull(rep_disposec0,''))+RTRIM(isnull(rep_disposec1,''))+RTRIM(isnull(rep_disposec2,'')) rep_disposec, \n [rep_reasond],\nRTRIM(rep_disposed)+RTRIM(isnull(rep_disposed0,''))+RTRIM(isnull(rep_disposed1,''))+RTRIM(isnull(rep_disposed2,'')) rep_disposed, \n[rep_reasone],\nRTRIM(rep_disposee)+RTRIM(isnull(rep_disposee0,''))+RTRIM(isnull(rep_disposee1,''))+RTRIM(isnull(rep_disposee2,'')) rep_disposee, \n [rep_reasonf],\nRTRIM(rep_disposef)+RTRIM(isnull(rep_disposef0,''))+RTRIM(isnull(rep_disposef1,''))+RTRIM(isnull(rep_disposef2,'')) rep_disposef\n,  [rep_remark1], [rep_remark3]\n  FROM ems.dbo.repair_hist \n  WHERE convert(varchar,rep_update1,111)=convert(varchar,getdate()-1,111)\n   and LEN(rtrim(rep_down_sites)) > 0 \n  and rep_deleted<>'Y' \n  union\n  SELECT [rep_machine], [rep_down_op],[rep_update1],  [rep_down_code], [rep_repair_op], [rep_update2], [rep_repair_op1], \n   [rep_update3],[rep_rc_no], \n  [rep_station], [rep_down_sites], \n  [rep_reason],[rep_dispose],  'NA' rep_reasona, 'NA' rep_disposea, 'NA' rep_reasonb,'NA' rep_disposeb, \n   'NA' rep_reasonc,'NA' rep_disposec, 'NA' rep_reasond, 'NA' rep_disposed, 'NA' rep_reasone, 'NA' rep_disposee,'NA' rep_reasonf, \n    'NA' rep_disposef , [rep_remark1], [rep_remark3]\n  FROM ems.dbo.repair_hist \n  WHERE convert(varchar,rep_update1,111)=convert(varchar,getdate()-1,111)\n   and LEN(rtrim(rep_down_sites)) = 0 \n  and rep_deleted<>'Y' \n  ORDER BY rep_machine,rep_update1 DESC", "connection reference"=w1495) -> ("error out"=w1490:errorcluster, "recordset reference"=w1494:T2)  [unwired: 5 in]
      n99 = call-poly <vilib>:"DB Tools Fetch Recordset Data.vi"("error in (no error)"=w1490, "recordset reference"=w1494) -> ("error out"=w1489:errorcluster, "recordset data"=w1436:variant[][], "recordset reference out"=w1493:T2)  [unwired: 3 in]
      n100 = Index Array(array=w1436, index (col) #1=0 ("index (row)"), index (col) #2=1 ("index (col)"), index (col) #3=2 ("disabled index (col)"), index (col) #4=3 ("index (col)"), index (col) #5=4 ("index (col)"), index (col) #6=5 ("index (col)"), index (col) #7=6 ("index (col)"), index (col) #8=7 ("index (col)"), index (col) #9=8 ("index (col)"), index (col) #10=9 ("index (col)"), index (col) #11=10 ("index (col)"), index (col) #12=11 ("index (col)"), index (col) #13=12 ("index (col)"), index (col) #14=13 ("index (col)"), index (col) #15=14 ("index (col)"), index (col) #16=15 ("index (col)"), index (col) #17=16 ("index (col)"), index (col) #18=17 ("index (col)"), index (col) #19=18 ("index (col)"), index (col) #20=19 ("index (col)"), index (col) #21=20 ("index (col)"), index (col) #22=21 ("index (col)"), index (col) #23=22 ("index (col)"), index (col) #24=23 ("index (col)"), index (col) #25=24 ("index (col)"), index (col) #26=25 ("index (col)"), index (col) #27=26 ("index (col)")) -> (element #1=w1465:variant[], element #2=w1464:variant[], element #3=w1476:variant[], element #4=w1475:variant[], element #5=w1474:variant[], element #6=w1473:variant[], element #7=w1472:variant[], element #8=w1471:variant[], element #9=w1470:variant[], element #10=w1469:variant[], element #11=w1468:variant[], element #12=w1467:variant[], element #13=w1449:variant[], element #14=w1448:variant[], element #15=w1447:variant[], element #16=w1446:variant[], element #17=w1445:variant[], element #18=w1444:variant[], element #19=w1443:variant[], element #20=w1442:variant[], element #21=w1441:variant[], element #22=w1440:variant[], element #23=w1439:variant[], element #24=w1438:variant[], element #25=w1437:variant[], element #26=w1432:variant[], element #27=w1429:variant[])  [unwired: 27 in]
      n101 = for {
        tunnel: w1476 -> [w1550] mode=indexing
        tunnel: w1475 -> [w1549] mode=indexing
        tunnel: w1474 -> [w1548] mode=indexing
        tunnel: w1473 -> [w1547] mode=indexing
        tunnel: w1472 -> [w1546] mode=indexing
        tunnel: w1471 -> [w1545] mode=indexing
        tunnel: w1470 -> [w1544] mode=indexing
        tunnel: w1469 -> [w1543] mode=indexing
        tunnel: w1468 -> [w1542] mode=indexing
        tunnel: w1467 -> [w1541] mode=indexing
        tunnel: [w1554] -> w1434
        shift-right: [w1554] -> _
        shift-left: string[][] [] ("array") -> [w1553]
        tunnel: w1465 -> [w1552] mode=indexing
        tunnel: w1464 -> [w1551] mode=indexing
        tunnel: w1449 -> [w1539] mode=indexing
        tunnel: w1448 -> [w1538] mode=indexing
        tunnel: w1447 -> [w1537] mode=indexing
        tunnel: w1446 -> [w1536] mode=indexing
        tunnel: w1445 -> [w1535] mode=indexing
        tunnel: w1444 -> [w1534] mode=indexing
        tunnel: w1443 -> [w1531] mode=indexing
        tunnel: w1442 -> [w1533] mode=indexing
        tunnel: w1441 -> [w1532] mode=indexing
        tunnel: w1440 -> [w1530] mode=indexing
        tunnel: w1439 -> [w1529] mode=indexing
        tunnel: w1438 -> [w1527] mode=indexing
        tunnel: w1437 -> [w1528] mode=indexing
        tunnel: w1432 -> [w1501] mode=indexing
        tunnel: w1429 -> [w1499] mode=indexing
        w1502 = ""
        n102 = xnode "Database Variant To Data"("database variant"=w1545, "type"=w1502) -> ("data"=w1520:string)  [unwired: 1 in, 1 out]
        n103 = xnode "Database Variant To Data"("database variant"=w1539, "type"=w1520) -> ("data"=w1517:string)  [unwired: 1 in, 1 out]
        n104 = xnode "Database Variant To Data"("database variant"=w1532, "type"=w1517) -> ("data"=w1509:string)  [unwired: 1 in, 1 out]
        n105 = xnode "Database Variant To Data"("database variant"=w1535, "type"=w1517) -> ("data"=w1513:string)  [unwired: 1 in, 1 out]
        n106 = xnode "Database Variant To Data"("database variant"=w1528, "type"=w1517) -> ("data"=w1498:string)  [unwired: 1 in, 1 out]
        "data" <- w1498
        n107 = xnode "Database Variant To Data"("database variant"=w1499, "type"=w1498) -> ("data"=w1497:string)  [unwired: 1 in, 1 out]
        n108 = xnode "Database Variant To Data"("database variant"=w1549, "type"=w1502) -> ("data"=w1526:string)  [unwired: 1 in, 1 out]
        n109 = xnode "Database Variant To Data"("database variant"=w1546, "type"=w1502) -> ("data"=w1523:string)  [unwired: 1 in, 1 out]
        n110 = xnode "Database Variant To Data"("database variant"=w1541, "type"=w1520) -> ("data"=w1518:string)  [unwired: 1 in, 1 out]
        n111 = xnode "Database Variant To Data"("database variant"=w1501, "type"=w1498) -> ("data"=w1500:string)  [unwired: 1 in, 1 out]
        n112 = xnode "Database Variant To Data"("database variant"=w1550, "type"=w1502) -> ("data"=w1505:string)  [unwired: 1 in, 1 out]
        n113 = xnode "Database Variant To Data"("database variant"=w1533, "type"=w1517) -> ("data"=w1510:string)  [unwired: 1 in, 1 out]
        n114 = xnode "Database Variant To Data"("database variant"=w1536, "type"=w1517) -> ("data"=w1514:string)  [unwired: 1 in, 1 out]
        n115 = xnode "Database Variant To Data"("database variant"=w1551, "type"=w1502) -> ("data"=w1503:string)  [unwired: 1 in, 1 out]
        n116 = xnode "Database Variant To Data"("database variant"=w1547, "type"=w1526) -> ("data"=w1524:string)  [unwired: 1 in, 1 out]
        n117 = xnode "Database Variant To Data"("database variant"=w1527, "type"=w1517) -> ("data"=w1506:string)  [unwired: 1 in, 1 out]
        n118 = xnode "Database Variant To Data"("database variant"=w1542, "type"=w1520) -> ("data"=w1519:string)  [unwired: 1 in, 1 out]
        n119 = xnode "Database Variant To Data"("database variant"=w1552, "type"=w1502) -> ("data"=w1504:string)  [unwired: 1 in, 1 out]
        "data 2" <- w1504
        n120 = xnode "Database Variant To Data"("database variant"=w1543, "type"=w1520) -> ("data"=w1521:string)  [unwired: 1 in, 1 out]
        n121 = xnode "Database Variant To Data"("database variant"=w1548, "type"=w1526) -> ("data"=w1525:string)  [unwired: 1 in, 1 out]
        n122 = xnode "Database Variant To Data"("database variant"=w1531, "type"=w1517) -> ("data"=w1511:string)  [unwired: 1 in, 1 out]
        n123 = xnode "Database Variant To Data"("database variant"=w1537, "type"=w1517) -> ("data"=w1515:string)  [unwired: 1 in, 1 out]
        n124 = xnode "Database Variant To Data"("database variant"=w1529, "type"=w1517) -> ("data"=w1507:string)  [unwired: 1 in, 1 out]
        n125 = xnode "Database Variant To Data"("database variant"=w1544, "type"=w1520) -> ("data"=w1522:string)  [unwired: 1 in, 1 out]
        n126 = xnode "Database Variant To Data"("database variant"=w1534, "type"=w1517) -> ("data"=w1512:string)  [unwired: 1 in, 1 out]
        n127 = xnode "Database Variant To Data"("database variant"=w1538, "type"=w1517) -> ("data"=w1516:string)  [unwired: 1 in, 1 out]
        n128 = xnode "Database Variant To Data"("database variant"=w1530, "type"=w1517) -> ("data"=w1508:string)  [unwired: 1 in, 1 out]
        n129 = Build Array(w1504, w1503, w1505, w1526, w1525, w1524, w1523, w1520, w1522, w1521, w1519, w1518, w1517, w1516, w1515, w1514, w1513, w1512, w1511, w1510, w1509, w1508, w1507, w1506, w1498, w1500, w1497) -> (w1540:string[])
        "appended array 4" <- w1540
        n130 = Insert Into Array(array=w1553, new element=w1540) -> (w1554:string[][])  [unwired: 2 in]
        "Value" <- w1528
      }
      n131 = call-poly <vilib>:"DB Tools Free Object.vi"("error in (no error)"=w1489, "recordset reference"=w1493) -> ("error out"=w1488:errorcluster, "connection reference"=w1492:T1)  [unwired: 8 in]
      n132 = call <vilib>:"DB Tools Close Connection.vi"("error in (no error)"=w1488, "connection reference"=w1492) -> ("error out"=→"error out 5":errorcluster)  [unwired: 5 in]
      n133 = local write "Table Control 3"(w1434) -> ()
    }
    frame #3 {
      w2426 = u16 1 items=["US", "Metric", "Default"] ("measurement system")
      w2436 = u16 1 items=["US", "Metric", "Default"] ("measurement system")
      w2447 = u16 1 items=["US", "Metric", "Default"] ("measurement system")
      w2448 = "E100Backup"
      w2462 = T3."Excel"  # Report Type
      # "Simulate UUT Testing"
      n134 = call <vilib>:"New Report.vi"("report type"=w2462, "template (empty)"="Report Template") -> ("report out"=w2459:refnum<class "NI_report.lvclass">, "error out"=w2458:errorcluster)  [unwired: 12 in]
      n135 = call <vilib>:"Excel Get Worksheet.vi"("report in"=w2459, "worksheet index (0)"=0, "error in (no error)"=w2458) -> ("report out"=w2453:refnum<class "NI_report.lvclass">, "error out"=w2452:errorcluster)  [unwired: 11 in]
      n136 = Get Date/Time In Seconds() -> (seconds since 1Jan1904=w2440:timestamp)
      n137 = call-poly <vilib>:"Append Table to Report.vi"("report in"=w2453, "column width (1)"=1.5, "measurement system"=w2447, "column headers"=string[] ["日期", "時間", "機台", "客戶", "使用時機\t", "使用檔名\t", "產品型號(光罩)\t", "設定溫度", "預熱秒數\t", "資料庫與出盤區設定\t", "空盤平移裝置(動作與位置)\t", "操作端吸嘴更換與吸取位置\t", "IC放置Shuttle定位\t", "IC運送梭Double Sensor\t", "Shuttle吸取釋放高度\t", "CCD影像反向測試\t", "Workpress及吸嘴吸取釋放動作正常\t", "測試端定位\t", "測試端高度校正\t", "出盤區定位\t", "測試區壓 測後檢查(1 EA/ Site)\t", "機板各部位接線確認\t", "改機人員\t", "確認者\t", "備註\n"] ("row headers"), "text data"="Table Control", "error in (no error)"=w2452) -> ("report out"=w2434:refnum<class "NI_report.lvclass">, "error out"=w2433:errorcluster)  [unwired: 6 in, 2 out]
      n138 = Get Date/Time String(seconds (now)=w2440) -> (date string=w2441:string)  [unwired: 2 in, 1 out]
      n139 = call <vilib>:"Excel Get Worksheet.vi"("report in"=w2434, "worksheet index (0)"=1, "error in (no error)"=w2433) -> ("report out"=w2438:refnum<class "NI_report.lvclass">, "error out"=w2437:errorcluster)  [unwired: 11 in]
      n140 = call-poly <vilib>:"Append Table to Report.vi"("report in"=w2438, "column width (1)"=1.5, "measurement system"=w2436, "column headers"=string[] ["Machine", "Customer", "Device", "Status", "Sites\t", "Code\t", "StartTime", "EndDate", "Time\t", "Operator\t", "FailSite", "Description\t", "Disposition\t"] ("row headers"), "text data"="Table Control 2", "error in (no error)"=w2437) -> ("report out"=w2424:refnum<class "NI_report.lvclass">, "error out"=w2423:errorcluster)  [unwired: 6 in, 2 out]
      n141 = call <vilib>:"Excel Get Worksheet.vi"("report in"=w2424, "worksheet index (0)"=2, "error in (no error)"=w2423) -> ("report out"=w2428:refnum<class "NI_report.lvclass">, "error out"=w2427:errorcluster)  [unwired: 11 in]
      n142 = call-poly <vilib>:"Append Table to Report.vi"("report in"=w2428, "column width (1)"=1.5, "measurement system"=w2426, "column headers"=string[] ["機台", "開單人", "開單時間", "代碼", "接單人\t", "接單時間\t", "結單人", "結單時間", "R/C #", "站點", "Sites\t", "原因", "處置\t", "原因A", "處置A", "原因B", "處置B", "原因C", "處置C", "原因D", "處置D", "原因E", "處置E", "原因F", "處置F", "開單備註\n", "結單備註"] ("row headers"), "text data"="Table Control 3", "error in (no error)"=w2427) -> ("report out"=w2422:refnum<class "NI_report.lvclass">, "error out"=w2421:errorcluster)  [unwired: 6 in, 2 out]
      n143 = Format Date/Time String(time format string (%c)="%Y%m%d%H", seconds (now)=w2440) -> (date/time string=w2445:string)  [unwired: 1 in]
      n144 = Concatenate Strings(w2448, w2445, ".xls" ("string")) -> (w2449:string)
      n145 = Concatenate Strings(w2448, w2445) -> ()  [unwired: 1 out]
      n146 = Build Path(base path=path "o:/monitor/E100backup", name or relative path=w2449) -> (appended path=w2443:path)
      n147 = call-dynamic "Save Report to File.vi"("report in"=w2422, "report file path"=w2443, "error in (no error)"=w2421) -> ("report out"=w2455:refnum<class "NI_report.lvclass">, "error out"=w2454:errorcluster)  [unwired: 11 in]
      n148 = call-dynamic "Dispose Report.vi"("report in"=w2455, "save changes? (F)"=FALSE, "error in (no error)"=w2454) -> ("error out"=→"error out 2":errorcluster)  [unwired: 12 in]
    }
    frame #4 {
      n149 = Index Array(array=w2465) -> (element=w2468:i32)  [unwired: 1 in]
      n150 = Greater?(x=w2468, y=1) -> (0:w2466:bool)
      n151 = case shown="True" w2466 {
        tunnel: w2464 -> [_ w2473]
        tunnel: w2463 -> [_ w2470]
        frame False {
        }
        frame True {
          (unwired) string[] ["yyliao@ptse.com.tw", "whlee@ptse.com.tw"] ("recipients")
          n152 = Concatenate Strings("***E100 Backup Data ***  " ("subject ([No Subject])"), w2470) -> (w2471:string)
          n153 = call <vilib>:"SMTP Email Send File.vi"("recipients"=string[] ["yyliao@ptse.com.tw"], "mail server"="192.168.1.17", "return address"="yyliao@ptse.com.tw", "subject ([No Subject])"=w2471, "message"="如附件", "file path"=w2473, "binary? (F)"=TRUE, "MIME content-type (application/octet-stream)"="application/octet-stream") -> ()  [unwired: 6 in, 2 out]
        }
      }
    }
    frame #5 {
      n154 = Quit LabVIEW() -> ()  [unwired: 1 in]
    }
  }
